vi "Enter_Drift_to_older_Calibs.vi"() -> ()   [LabVIEW 2010]
uses:
  Controls/Cal_Inst_type.ctl
panel:
  in  "Instrument type":T1=enum."Cross wire velocity"
  in  "Calib file Orig":path=path "/iMac_3 HD/Users/Hong(6%)/calib/XW Ch 1 7_10_02_5"
  in  "Calib file New":path=path "/iMac_3 HD/Users/Hong(6%)/calib/XW Ch 1 7_10_02_6"
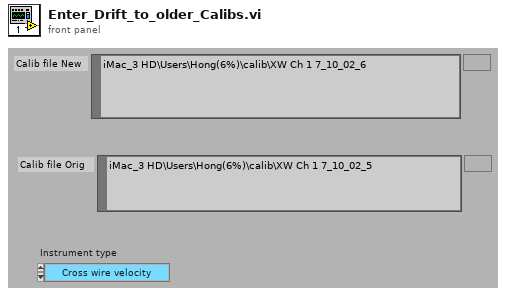
[diagram p1: front panel]
types:
  T1 = typedef "Cal_Inst_type.ctl" = enum16{"Propeller anemometer", "Pressure Transducer", "Hot wire", "Cross wire velocity", "Cross wire angle", "Generic Linear", "Generic Polynomial", "Generic BackPoly", "Fast FID", "Thermocouple", "Cold wire", "Pulsed Wire"}
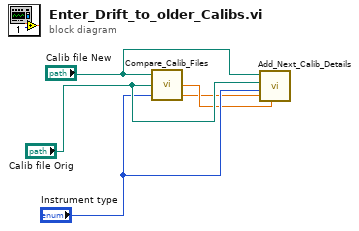
[diagram p0: block diagram]
diagram:
  n1 = call "Compare_Calib_Files.vi"("Instrument type"="Instrument type", "Calib file Orig"="Calib file Orig", "Calib file New"="Calib file New") -> ("Calib Time Separation (Hours)"=w1:dbl, "% Change"=w2:dbl)  [unwired: 1 out]
  n2 = call "Add_Next_Calib_Details.vi"("% Change"=w2, "Hours between calibrations"=w1, "Instrument type"="Instrument type", "Calib file Orig"="Calib file Orig", "Calib file New"="Calib file New") -> ()  [unwired: 1 in, 1 out]
